vi "Read from Hardware.vi"(8 "error in":errorcluster, 10 "values in":dbl[](array[numeric]), 11 "Rx execution unit in":refnum<class "Rx Execution Unit.lvclass">) -> (0 "error out":errorcluster, 2 "values out":dbl[](array[numeric]), 3 "Rx execution unit out":refnum<class "Rx Execution Unit.lvclass">)   [LabVIEW 2020, in "Ballard MIL-STD-1553 Engine.lvlib" / "Implementation.lvlib" / "Rx Execution Unit.lvclass"]
uses:
  Rx Execution Unit.lvclass
  C:/dev/niveristand-ballard-milStd1553-custom-device/Source/Custom Device Support/Engine/Implementation/Execution Unit/Execution Unit.lvclass
  Rx Execution Unit.lvclass/Rx Execution Unit.ctl
  Custom Device/Write Error to System Log.vi/ca55ed61-c1f5-4d13-8aef-490b87d2cf89.vi
  <vilib>/NI VeriStand/Custom Device Tools/Custom Device Utility Library/NI VeriStand - Print Debug Line.vi
  Execution Unit/Execution Unit.lvclass
  Custom Device/Custom Device.lvlib
  <instrlib>/BTI1553Lib/BTI1553LV.lvlib
  C:/dev/niveristand-ballard-milStd1553-custom-device/Source/Custom Device Support/Engine/Interfaces/Execution Unit/Execution Unit.lvclass
  C:/dev/niveristand-ballard-milStd1553-custom-device/Source/Custom Device Support/Engine/Implementation/Rx Execution Unit/Rx Execution Unit.lvclass
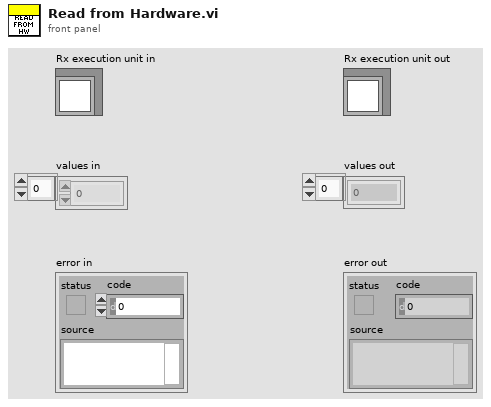
[diagram p1: front panel]
types:
  T1 = typedef "Rx Read Info.ctl" = cluster{"transfer handle":u64, "terminal address":u16}
  T2 = typedef "BTI1553LV.lvlib/1553 Message Fields.ctl" = cluster{"msgflag":u16, "msgopt":u16, "anyerror":bool, "noresponse":bool, "allretriesfailed":bool, "protocolerror":bool, "wrongsyncerror":bool, "datacounterror":bool, "manchestererror":bool, "parityerror":bool, "worderror":bool, "systemerror":bool, "hit":bool, "reserved":u8, "channelnumber":i32, "transmittedcwd1":bool, "transmittedcwd2":bool, "transmittedswd1":bool, "transmittedswd2":bool, "receivedcwd1":bool, "receivedcwd2":bool, "receivedswd1":bool, "receivedswd2":bool, "transmitteddwd":bool, "receiveddwd":bool, "reserved":i8, "reserved":i8, "bus":u32, "resptime1":u16, "resptime2":u16, "datacount":u16, "extflag":u16, "timetagh":u32, "timetag_hitcount":u32, "elapsetime_mintime_maxtime":u32, "cwd1":u16, "cwd2":u16, "swd1":u16, "swd2":u16, "data":u16[], "extra":u16[]}
  T3 = typedef "Ballard MIL-STD-1553 Engine.lvlib/Implementation.lvlib/Rx Execution Unit.lvclass/Status Error Counts.ctl" = cluster{"general protocol error count":u64, "improper number of words error count":u64, "manchester error count":u64, "monitor error count":u64, "parity error count":u64, "unconfigured frames error count":u64, "word error count":u64, "wrong sync error count":u64}
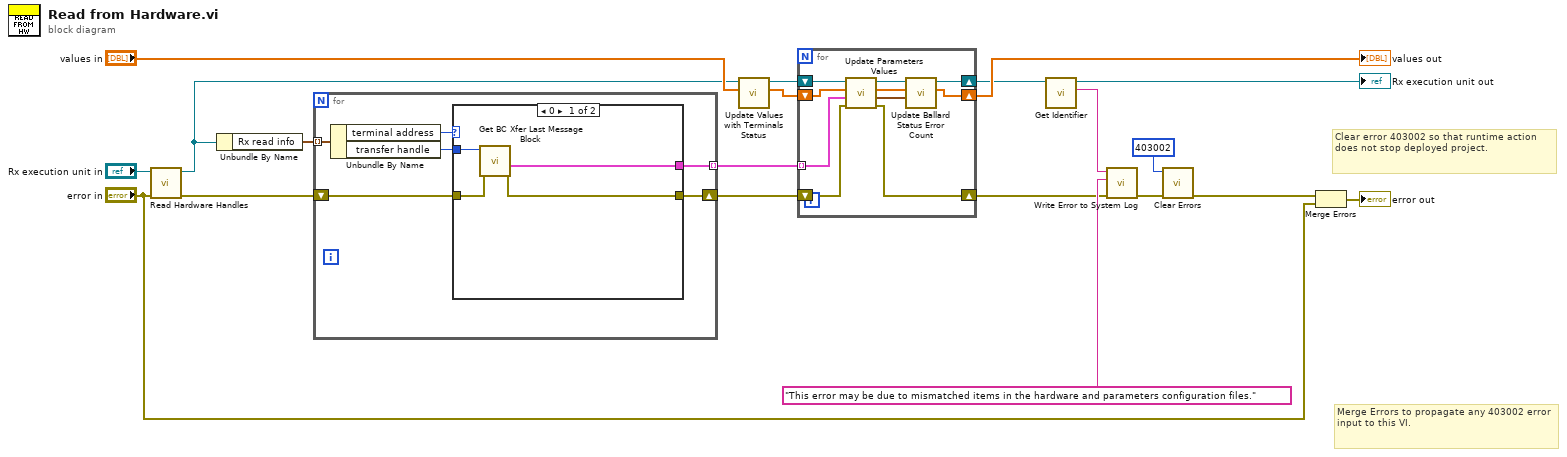
[diagram p0: block diagram]
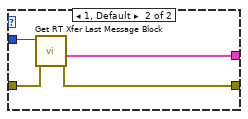
[diagram p2: hidden frame]
diagram:
  # "Clear error 403002 so that runtime action does not stop deployed project."
  # "Merge Errors to propagate any 403002 error input to this VI."
  n1 = call "Read Hardware Handles.vi"("error in"="error in", "Execution Unit in"="Rx execution unit in") -> ("error out"=w2:errorcluster, "Execution Unit out"=w6:refnum<class "Rx Execution Unit.lvclass">)  [unwired: 7 in, 1 out]
  n2 = Unbundle By Name(w6) -> ("Rx read info"=w5:T1[])
  n3 = for {
    tunnel: w5 -> [w26] mode=indexing
    shift-right: [w21] -> w1
    shift-left: w2 -> [w22]
    tunnel: [w25] -> w4 mode=indexing
    n4 = Unbundle By Name(w26) -> ("terminal address"=w24:u16, "transfer handle"=w23:u64)
    n5 = case shown="0" w24 {
      tunnel: w23 -> [w28 w34]
      tunnel: w22 -> [w30 w33]
      tunnel: [w27 w31] -> w21
      tunnel: [w29 w32] -> w25
      frame 0 {
        n6 = call <instrlib>:"Get BC Xfer Last Message Block.vi"("error in (no error)"=w30, "bc transfer handle in"=w28) -> ("error out"=w27:errorcluster, "message fields out"=w29:T2)  [unwired: 6 in, 2 out]
      }
      frame 1, Default {
        n7 = call <instrlib>:"Get RT Xfer Last Message Block.vi"("error in (no error)"=w33, "rt transfer handle in"=w34) -> ("error out"=w31:errorcluster, "message fields out"=w32:T2)  [unwired: 6 in, 2 out]
      }
    }
  }
  n8 = call "Update Values with Terminals Status.vi"("values in"="values in", "Rx execution unit in"=w6) -> ("values out"=w8:dbl[], "Rx execution unit out"=w9:refnum<class "Rx Execution Unit.lvclass">)  [unwired: 7 in, 1 out]
  n9 = for {
    shift-right: [w36] -> w3
    shift-left: w1 -> [w41]
    shift-right: [w42] -> w20
    shift-left: w8 -> [w44]
    shift-right: [w43] -> w7
    shift-left: w9 -> [w38]
    tunnel: w4 -> [w35] mode=indexing
    n10 = call "Update Parameters Values.vi"("error in"=w41, "message fields"=w35, "values in"=w44, "Rx execution unit in"=w38) -> ("error out"=w36:errorcluster, "status error counts"=w40:T3, "values out"=w39:dbl[], "Rx execution unit out"=w37:refnum<class "Rx Execution Unit.lvclass">)  [unwired: 4 in]
    n11 = call "Update Ballard Status Error Count.vi"("status error counts"=w40, "values in"=w39, "Rx execution unit in"=w37) -> ("values out"=w42:dbl[], "Rx execution unit out"=w43:refnum<class "Rx Execution Unit.lvclass">)  [unwired: 7 in]
  }
  "values out" <- w20
  n12 = call-dynamic "Get Identifier.vi"("Execution Unit Implementation in"=w7) -> ("Identifier"=w14:string, "Execution Unit Implementation out"=→"Rx execution unit out":refnum<class "Rx Execution Unit.lvclass">)  [unwired: 8 in, 1 out]
  n13 = call "Write Error to System Log.vi"("error in"=w3, "message"="This error may be due to mismatched items in the hardware and parameters configuration files.", "identifier"=w14) -> ("error out"=w13:errorcluster)  [unwired: 8 in]
  n14 = call <vilib>:"Clear Errors.vi"("error in (no error)"=w13, "specific error code to clear (0: all)"=403002) -> ("error out"=w16:errorcluster)  [unwired: 4 in, 1 out]
  n15 = Merge Errors(w16, "error in") -> (→"error out":errorcluster)
